vi "ExCustomTiming.vi"(1 "error in (no error)":errorcluster, 2 "Vertical timing":dbl=30.2) -> (0 "error out":errorcluster)   [LabVIEW 2010]
uses:
  Users/Public/Documents/SItoolkit/LabVIEW/Examples2010_5_0_0_0/Fast Examples/Open-Close Hardware/CamHandle.vi
panel:
  out "Vertical timing returned":dbl
  # "ExCustomTiming.vi : this allows the vertical \ntiming register to be set, This is a floating point\nvalue. this is new to 64 bits, it use to be index"
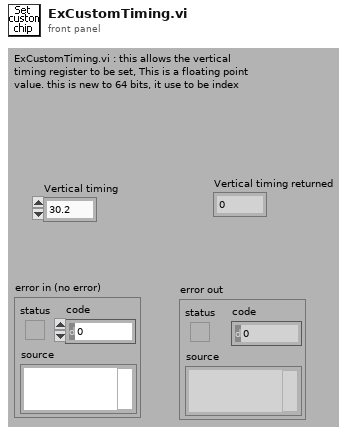
[diagram p1: front panel]
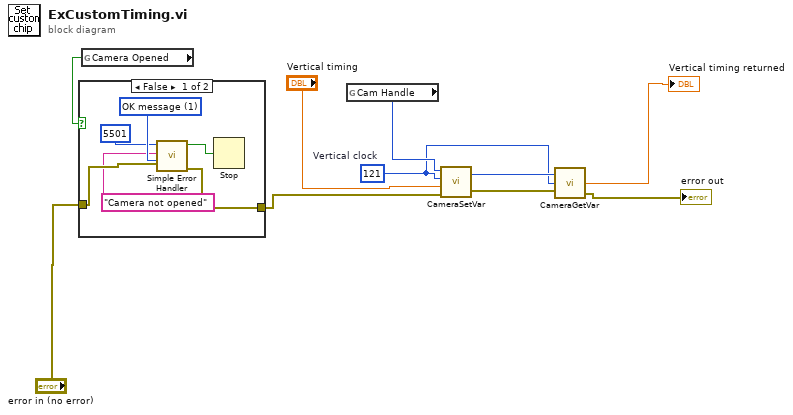
[diagram p0: block diagram]
diagram:
  w4 = u32 121  # Vertical clock
  n1 = global read "CamHandle.vi" "Camera Opened"() -> (w10:bool)
  n2 = case shown="False" w10 {
    tunnel: "error in (no error)" -> [w15 w17]
    tunnel: [w14 w17] -> w8
    frame False {
      w16 = u16 1 items=["no dialog", "OK message", "continue or stop message"] ("type of dialog (OK msg:1)")
      n3 = call <vilib>:"Simple Error Handler.vi"("error code (no error:0)"=5501, "error source (\" \")"="Camera not opened", "type of dialog (OK msg:1)"=w16, "error in (no error)"=w15) -> ("error?"=w12:bool, "error out"=w14:errorcluster)  [unwired: 1 in, 3 out]
      n4 = Stop(stop? (T)=w12) -> ()
    }
    frame True {
    }
  }
  n5 = global read "CamHandle.vi" "Cam Handle"() -> (w6:u32)
  n6 = call <userlib>:"CameraSetVar.vi"("error in"=w8, "Value"="Vertical timing", "Parameter ID"=w4, "Camera Handle"=w6) -> ("error out"=w3:errorcluster, "CameraHandle"=w5:u32)
  n7 = call <userlib>:"CameraGetVar.vi"("error in"=w3, "Parameter ID"=w4, "Camera Handle"=w5) -> ("error out"=→"error out":errorcluster, "Value"=→"Vertical timing returned":dbl)  [unwired: 1 out]
